vi "PWM Waveform PD250 Test.vi"(0 "Analysis Leg":i32, 1 "Board Selector":T2, 5 "Active Leg":i32, 9 "Waveform":waveform(dbl)[](array[waveform])) -> (4 "Inactive Values":T1, 6 "Active Values":T1, 15 "error out":errorcluster)   [LabVIEW 2022 SP3]
uses:
  Serial Board Com/Board Select.ctl
  <vilib>/Analysis/Matrix/Datatypes/RealMatrix.ctl
  <vilib>/measure/mascope.llb/Pulse Measurements 1 chan.vi
  <vilib>/measure/madcrms.llb/Basic Averaged DC-RMS for 1 Chan.vi
  <vilib>/measure/NI_MAPro.lvlib
  <vilib>/Analysis/Matrix/NI_Matrix.lvlib
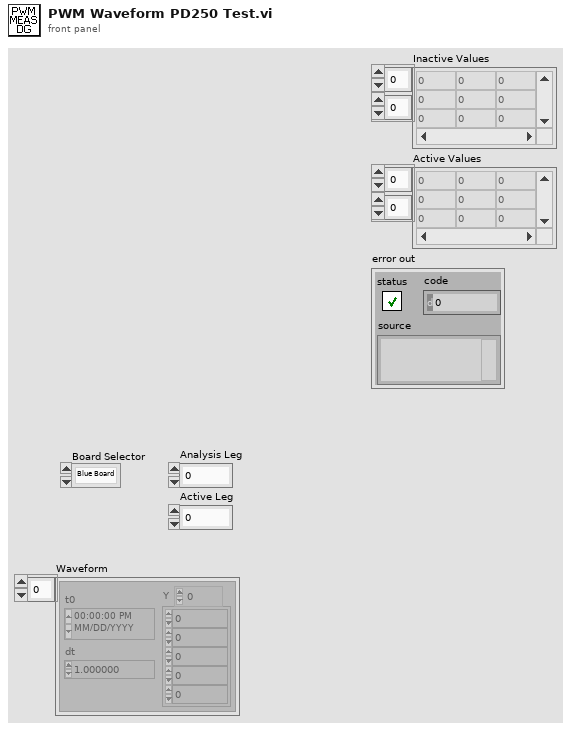
[diagram p1: front panel]
types:
  T1 = typedef "NI_Matrix.lvlib/RealMatrix.ctl" = dbl[][]
  T2 = typedef "Board Select.ctl" = enum16{"Blue Board", "Green Board"}
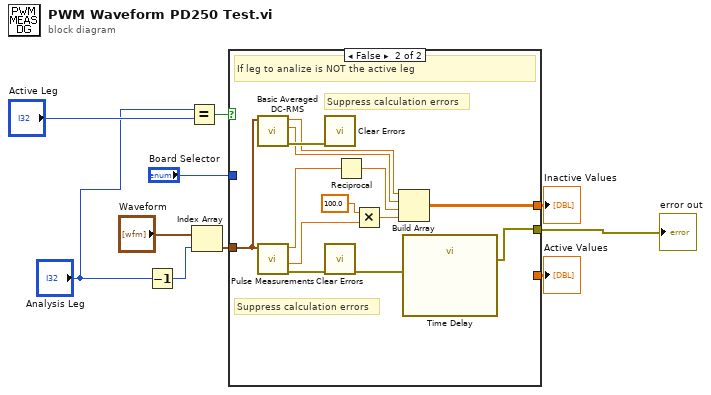
[diagram p0: block diagram]
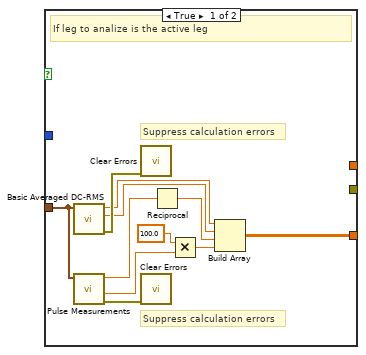
[diagram p2: hidden frame]
diagram:
  n1 = Decrement(x="Analysis Leg") -> (x-1=w1:i32)
  n2 = Equal?(x="Analysis Leg", y="Active Leg") -> (x = y?=w8:bool)
  n3 = Index Array(array="Waveform", index=w1) -> (element=w9:waveform(dbl))
  n4 = case shown="False" w8 {
    tunnel: w9 -> [w16 w29]
    tunnel: "Board Selector" -> [_ _]
    tunnel: [_ w24] -> w6
    tunnel: [w11 _] -> w5
    tunnel: [_ w22] -> w3
    frame True {
      # "Suppress calculation errors"
      # "Suppress calculation errors"
      # "If leg to analize is the active leg"
      n5 = call-poly <vilib>:"Basic Averaged DC-RMS.vi"("signal in"=w16) -> ("error out"=w17:errorcluster, "RMS value"=w14:dbl, "DC value"=w15:dbl)  [unwired: 7 in, 1 out]
      n6 = call-poly <vilib>:"Pulse Measurements.vi"("signal in"=w16) -> ("error out"=w18:errorcluster, "duty cycle"=w20:dbl, "period"=w19:dbl)  [unwired: 6 in, 2 out]
      n7 = call <vilib>:"Clear Errors.vi"("error in (no error)"=w17) -> ()  [unwired: 5 in, 2 out]
      n8 = call <vilib>:"Clear Errors.vi"("error in (no error)"=w18) -> ()  [unwired: 5 in, 2 out]
      n9 = Reciprocal(x=w19) -> (1/x=w13:dbl)
      n10 = Multiply(x=100.0, y=w20) -> (x*y=w12:dbl)
      n11 = Build Array(w15, w14, w13, w12) -> (w11:T1)
    }
    frame False {
      # "Suppress calculation errors"
      # "Suppress calculation errors"
      # "If leg to analize is NOT the active leg"
      n12 = call-poly <vilib>:"Basic Averaged DC-RMS.vi"("signal in"=w29) -> ("error out"=w30:errorcluster, "RMS value"=w27:dbl, "DC value"=w28:dbl)  [unwired: 7 in, 1 out]
      n13 = call-poly <vilib>:"Pulse Measurements.vi"("signal in"=w29) -> ("error out"=w31:errorcluster, "duty cycle"=w33:dbl, "period"=w32:dbl)  [unwired: 6 in, 2 out]
      n14 = call <vilib>:"Clear Errors.vi"("error in (no error)"=w30) -> ()  [unwired: 5 in, 2 out]
      n15 = call <vilib>:"Clear Errors.vi"("error in (no error)"=w31) -> ("error out"=w23:errorcluster)  [unwired: 5 in, 1 out]
      n16 = Reciprocal(x=w32) -> (1/x=w26:dbl)
      n17 = Multiply(x=100.0, y=w33) -> (x*y=w25:dbl)
      n18 = Build Array(w28, w27, w26, w25) -> (w24:T1)
      n19 = call "Time Delay"("error in (no error)"=w23) -> ("error out"=w22:errorcluster)  [unwired: 10 in]
    }
  }
  "Inactive Values" <- w6
  "Active Values" <- w5
  "error out" <- w3
